vi "Boolean Control - Boolean Button Timed.vi"() -> ()   [LabVIEW 2014]
doc: "Sample numeric display item."
uses:
  <vilib>/NI Veristand/Display Template Support/Display Template Support.llb/cluster_Screen Item Settings.ctl
  <vilib>/NI Veristand/Display Template Support/Display Template Support.llb/cluster_Graph Scale Settings.ctl
  <vilib>/NI Veristand/Display Template Support/Display Template Support.llb/cluster_Graph Plot Settings.ctl
  SubVIs/Boolean Control Timed.ctl
  NationalInstruments.VeriStand.SystemStorage
  <vilib>/NI Veristand/Display Template Support/Display Template Support.llb/enum_Display Template Handler Minimal To Widget Msg.ctl
  <vilib>/NI Veristand/Display Template Support/Display Template Support.llb/enum_Display Template Handler Minimal To Workspace.ctl
  SubVIs/Boolean Control Timed Data.ctl
  <vilib>/NI Veristand/Display Template Support/Display Template Support.llb/sub_Display Template Handler Custom.vi
  <vilib>/NI Veristand/Execution/Workspace/NI VeriStand - Set Single Channel Value.vi
  <vilib>/NI Veristand/Execution/Workspace/NI VeriStand - Get Single Channel Value.vi
  <vilib>/NI Veristand/Execution/Workspace/NI_VS Workspace ExecutionAPI.lvlib
panel:
  in  "NIVS.System Definition Root":refnum<k24>
  in  "NIVS.Gateway IP Address":string
  out "Label":string="Numeric"
  in  "Boolean Timed":T1
  in  "Item.Data":T2
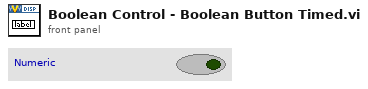
[diagram p1: front panel]
types:
  T1 = typedef "Boolean Control Timed.ctl" = bool
  T2 = typedef "cluster_Screen Item Settings.ctl" = cluster{"Template VI":string, "Position X":i32, "Position Y":i32, "Custom":string, "Show Title Bar":bool, "ID":i32, "Always On Top":bool, "Allow Resize":bool, "Allow Minimize":bool, "Allow Close":bool, "Size to Screen":bool, "Screen.ID":i32, "State":enum16{"Normal", "New"}, "Title":string, "Window Bounds":cluster{"[0]":i16, "[1]":i16, "[2]":i16, "[3]":i16}, "Channel Ref":u64, "Unit":string, "Default Units?":bool, "Flash Limit?":bool, "Color 1":u32, "Color 2":u32, "Color 3":u32, "Color 4":u32, "Bck Color":u32, "Fore Color":u32, "Limit 1":dbl, "Limit 2":dbl, "Limit 3":dbl, "Limit 4":dbl, "Limit Mode 1":i32, "Limit Mode 2":i32, "Limit Mode 3":i32, "Limit Mode 4":i32, "Scale Precision":i32, "Scale Min":dbl, "Scale Max":dbl, "Format":i32, "Precision":i32, "Background Type":i32, "IDs":i32[], "Units":string[], "Labels":string[], "Scale Factor":dbl, "Scale Offset":dbl, "YScale Index":u32[], "XScale":T3, "YScales":T3[], "Plots":T4[], "Update Period":dbl, "History Length":dbl, "My.Ref":refnum<vi>, "Is Control?":bool, "Channel Paths":string[], "Custom Data":variant}
  T3 = typedef "cluster_Graph Scale Settings.ctl" = cluster{"Format":u8, "Precision":u8, "Fit":u8, "Label":string, "Use Default Label":bool, "Label Visible":bool, "Min":dbl, "Max":dbl}
  T4 = typedef "cluster_Graph Plot Settings.ctl" = cluster{"Bar Style":u8, "Fill To":i16, "Fill/PtColor":u32, "Line Style":u8, "Line Width":u8, "Color":u32, "Interp":u8, "Point Style":u8}
  T5 = cluster{"Timer Running?":bool, "Initial Time":u32}
  T6 = typedef "enum_Display Template Handler Minimal To Workspace.ctl" = cluster{"Operation":enum16{"SetCustomData", "DeleteItem"}, "Data":variant}
  T7 = typedef "enum_Display Template Handler Minimal To Widget Msg.ctl" = enum16{"Stop", "LaunchConfigDialog"}
  T8 = typedef "Boolean Control Timed Data.ctl" = cluster{"Node Path":string, "Time (ms)":u32}
  T9 = typedef "NI_VS Workspace ExecutionAPI.lvlib/WorkspaceAPI.ctl" = refnum<k24>
  T10 = typedef "NI_VS Workspace ExecutionAPI.lvlib/SystemState.ctl" = u8
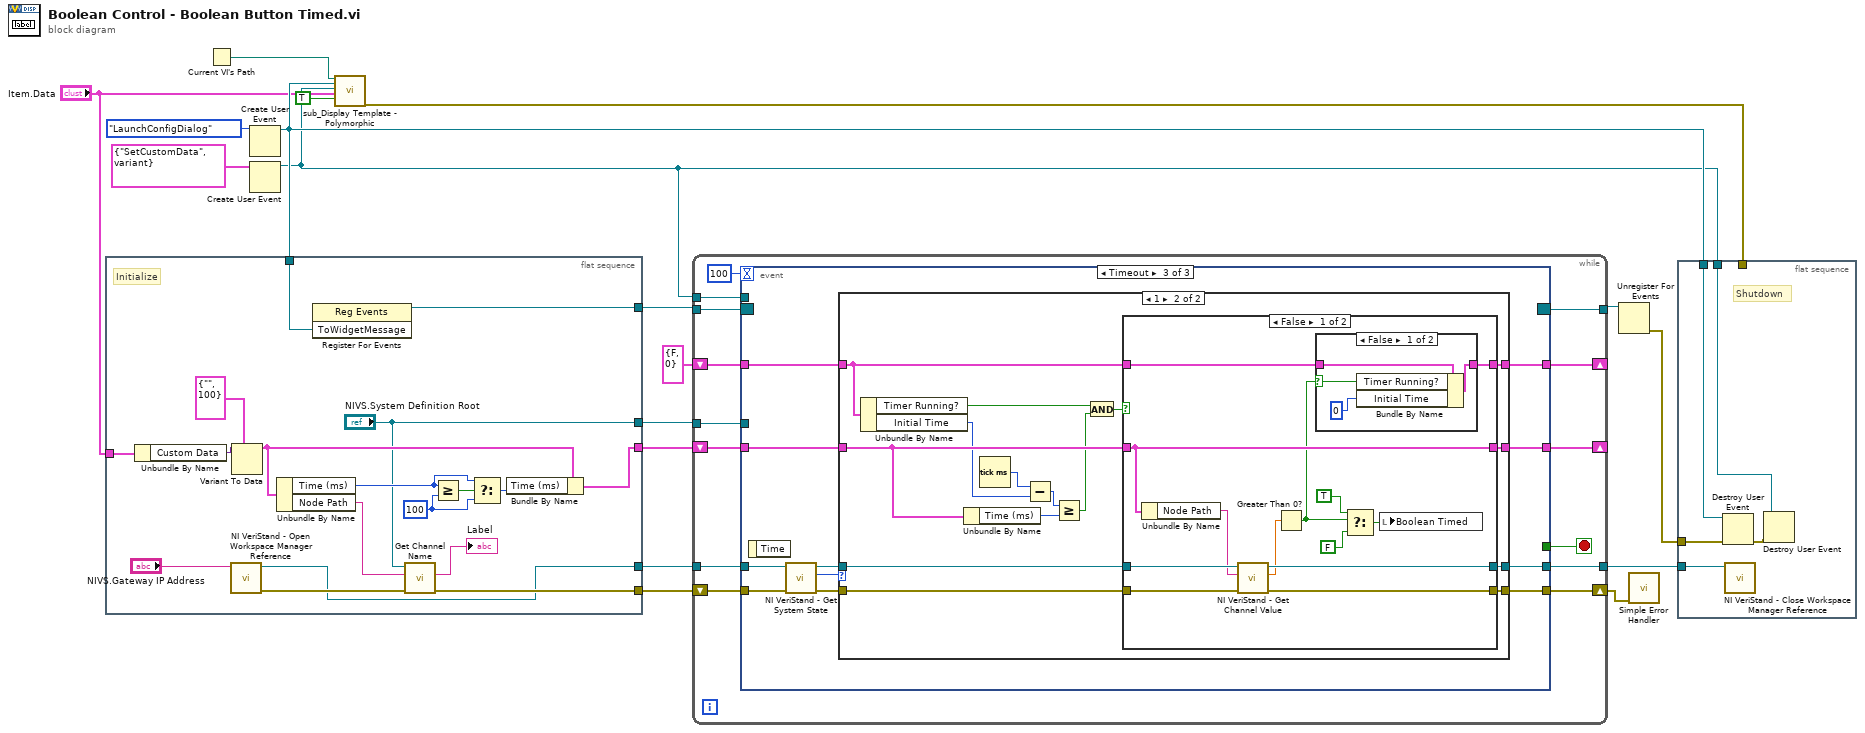
[diagram p0: block diagram]
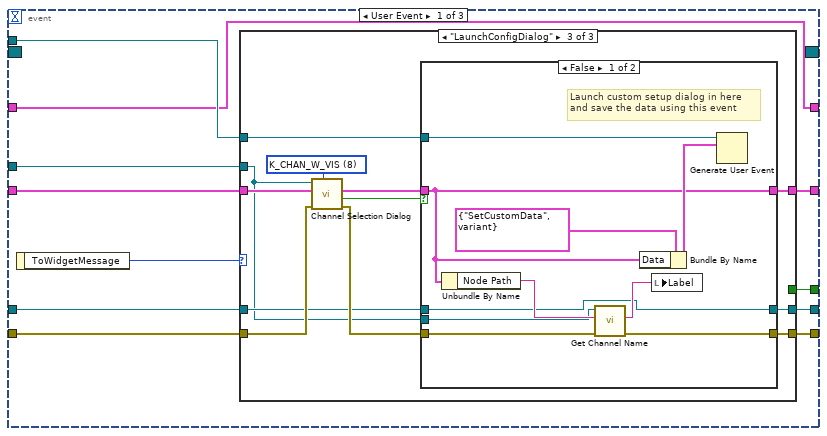
[diagram p2: hidden frame]
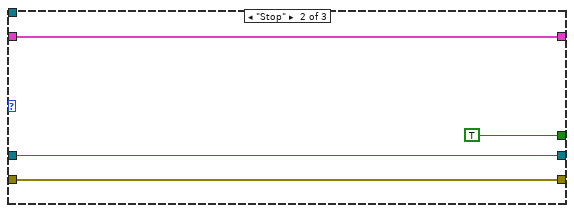
[diagram p4: hidden frame]
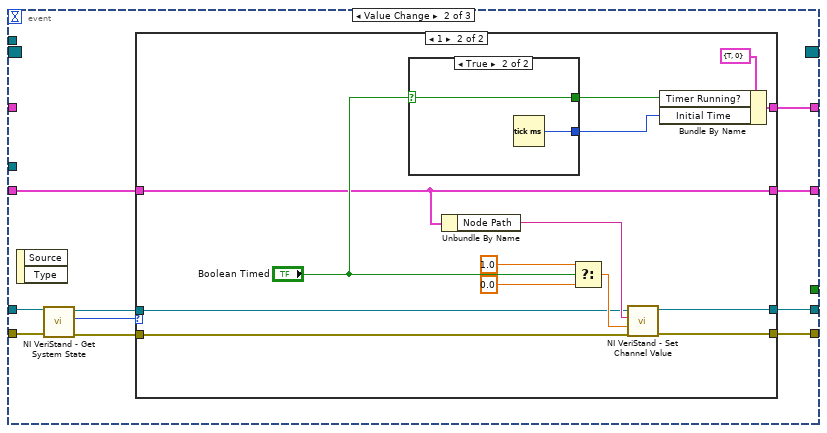
[diagram p6: hidden frame]
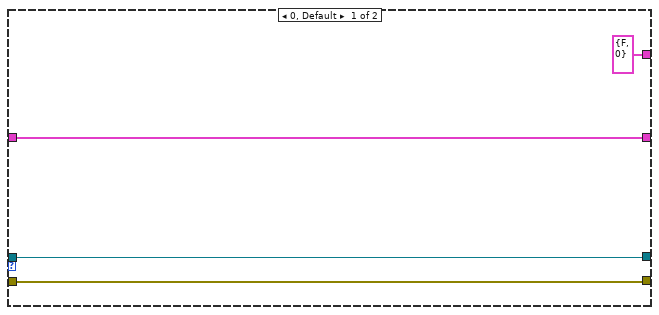
[diagram p7: hidden frame]
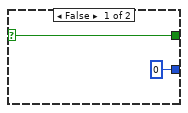
[diagram p8: hidden frame]
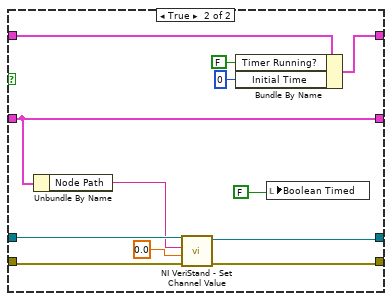
[diagram p11: hidden frame]
diagram:
  n1 = flat-sequence {
    tunnel: [w36] -> w16
    tunnel: w13 -> [w35]
    tunnel: "Item.Data" -> [w34]
    tunnel: [w21] -> w7
    tunnel: [w19] -> w4
    tunnel: [w29] -> w5
    tunnel: ["NIVS.System Definition Root"] -> w6
    frame #0 {
      w23 = u32 100 ("y")
      # "Initialize"
      n2 = Unbundle By Name(w34) -> ("Custom Data"=w33:variant)
      n3 = call <vilib>:"NI VeriStand - Open Workspace Manager Reference.vi"("Gateway IP Address (\"\": localhost)"="NIVS.Gateway IP Address") -> ("error out"=w31:errorcluster, "WorkspaceManager"=w19:T9)  [unwired: 9 in]
      n4 = Variant To Data(type=T8 {"Node Path"="", "Time (ms)"=100}, Variant=w33) -> (data=w26:T8)  [unwired: 1 in, 1 out]
      n5 = Unbundle By Name(w26) -> ("Time (ms)"=w24:u32, "Node Path"=w27:string)
      n6 = register-events(w35) -> (reference out=w36:refnum<event-registration>)  [unwired: 2 in, 1 out]
      n7 = call "Get Channel Name.vi"("error in (no error)"=w31, "Node Path"=w27, "NIVS.System Definition Root in"="NIVS.System Definition Root") -> ("error out"=w29:errorcluster, "Name"=→"Label":string)  [unwired: 6 in, 1 out]
      n8 = Greater Or Equal?(x=w24, y=w23) -> (x >= y?=w25:bool)
      n9 = Select(t=w24, s=w25, f=w23) -> (s? t:f=w22:u32)
      n10 = Bundle By Name(cluster=w26, "Time (ms)"=w22) -> (w21:T8)
    }
  }
  n11 = Current VI's Path() -> (path=w11:path)
  n12 = Create User Event(user event datatype=enum_Display_Template_Handler_Minimal_To_Widget_Msg."LaunchConfigDialog" ("ToWidgetMessage")) -> (user event=w13:refnum<user-event>)  [unwired: 1 in, 1 out]
  n13 = Create User Event(user event datatype=T6 {"Operation"=enum."SetCustomData", "Data"=variant} ("Data")) -> (user event=w9:refnum<user-event>)  [unwired: 1 in, 1 out]
  n14 = call-poly <vilib>:"sub_Display Template - Polymorphic.vi"("Parent.Path"=w11, "ToWidgetEvent"=w13, "ToWorkspace"=w9, "Item.Data"="Item.Data", "Resizable"=TRUE) -> ("error out"=w18:errorcluster)  [unwired: 1 in, 13 out]
  n15 = while {
    tunnel: w16 -> [w50]
    tunnel: [w48] -> w15
    tunnel: w9 -> [w47]
    shift-right: [w40] -> _
    shift-left: w7 -> [w46]
    tunnel: w6 -> [w45]
    shift-right: [w42] -> w1
    shift-left: w5 -> [w44]
    tunnel: w4 -> [w43]
    tunnel: [w41] -> w3
    shift-right: [w38] -> _
    shift-left: T5 {"Timer Running?"=FALSE, "Initial Time"=0} -> [w37]
    stop <- w49 stop-if-true
    n16 = event shown="[2] Timeout" {
      selector: w50 -> [_ _ _]
      dyn-events: [_ _ _] -> w48
      timeout: 100 -> [_ _ _]
      tunnel: [w60 _ _] -> w49
      tunnel: w47 -> [w59 _ _]
      tunnel: w46 -> [w58 w101 w132]
      tunnel: w45 -> [w57 _ _]
      tunnel: w44 -> [w56 w98 w129]
      tunnel: w43 -> [w55 w99 w130]
      tunnel: [w54 w103 w136] -> w42
      tunnel: [w53 w102 w135] -> w41
      tunnel: [w52 w94 w134] -> w40
      tunnel: [w51 w100 w131] -> w38
      tunnel: w37 -> [w51 _ w133]
      event User Event {
        n17 = event-data() -> ("ToWidgetMessage"=w61:T7)  [unwired: 1 out]
        n18 = case shown="\"LaunchConfigDialog\"" w61 {
          tunnel: [_ TRUE _] -> w60
          tunnel: w59 -> [_ _ w80]
          tunnel: w58 -> [w62 w65 w78]
          tunnel: w57 -> [_ _ w69]
          tunnel: w56 -> [w64 w67 w77]
          tunnel: w55 -> [w63 w66 w73]
          tunnel: [w64 w67 w72] -> w54
          tunnel: [w63 w66 w71] -> w53
          tunnel: [w62 w65 w70] -> w52
          frame Default {
          }
          frame "Stop" {
          }
          frame "LaunchConfigDialog" {
            w79 = u8 8 items=["K_CHAN_R", "K_CHAN_W", "K_CHAN_RW", "K_CHAN_VOLT", "K_CHAN_FAULT", "K_ALL", "K_CUSTOM", "K_CHAN_R_VIS", "K_CHAN_W_VIS", "K_CHAN_RW_VIS", "K_CHAN_VOLT_VIS", "K_CHAN_FAULT_VIS"] ("DisplayFilter")
            n19 = call "Channel Selection Dialog.vi"("DisplayFilter"=w79, "error in (no error)"=w77, "Custom Data in"=w78, "NIVS.System Definition Root"=w69) -> ("error out"=w74:errorcluster, "Cancelled"=w76:bool, "Custom Data out"=w75:T8)  [unwired: 5 in]
            n20 = case shown="False" w76 {
              tunnel: w80 -> [w90 _]
              tunnel: w75 -> [w84 w91]
              tunnel: w74 -> [w86 w92]
              tunnel: w73 -> [w82 w93]
              tunnel: [w85 w92] -> w72
              tunnel: [w82 w93] -> w71
              tunnel: [w84 w91] -> w70
              tunnel: w69 -> [w81 _]
              frame False {
                # "Launch custom setup dialog in here\nand save the data using this event"
                n21 = Unbundle By Name(w84) -> ("Node Path"=w83:string)
                n22 = call "Get Channel Name.vi"("error in (no error)"=w86, "Node Path"=w83, "NIVS.System Definition Root in"=w81) -> ("error out"=w85:errorcluster, "Name"=w87:string)  [unwired: 6 in, 1 out]
                n23 = Bundle By Name(cluster=T6 {"Operation"=enum."SetCustomData", "Data"=variant} ("event data"), "Data"=w84) -> (w88:T6)
                n24 = local write "Label"(w87) -> ()
                n25 = Generate User Event(user event=w90, event data cluster=w88) -> ()  [unwired: 2 in, 2 out]
              }
              frame True {
              }
            }
          }
        }
      }
      event Value Change {
        n26 = event-data() -> ()  [unwired: 3 out]
        n27 = call <vilib>:"NI VeriStand - Get System State.vi"("error in (no error)"=w98, "WorkspaceManager in"=w99) -> ("error out"=w97:errorcluster, "System State"=w95:T10, "WorkspaceManager  out"=w96:T9)  [unwired: 5 in, 2 out]
        n28 = case shown="1" w95 {
          tunnel: [w107 w121] -> w103
          tunnel: [w106 w120] -> w102
          tunnel: w101 -> [w105 w108]
          tunnel: [T5 {"Timer Running?"=FALSE, "Initial Time"=0} w111] -> w100
          tunnel: w97 -> [w107 w110]
          tunnel: w96 -> [w106 w109]
          tunnel: [w105 w108] -> w94
          frame 0, Default {
          }
          frame 1 {
            n29 = case shown="True" "Boolean Timed" {
              selector: "Boolean Timed" -> [w123 w125]
              tunnel: [w123 w125] -> w113
              tunnel: [u32 0 ("millisecond timer value") w124] -> w112
              frame False {
              }
              frame True {
                n30 = Tick Count (ms)() -> (millisecond timer value=w124:u32)
              }
            }
            n31 = Unbundle By Name(w108) -> ("Node Path"=w116:string)
            n32 = Select(t=1.0, s="Boolean Timed", f=0.0) -> (s? t:f=w117:dbl)
            n33 = call-poly <vilib>:"NI VeriStand - Set Channel Value.vi"("error in (no error)"=w110, "Value"=w117, "Channel"=w116, "WorkspaceManager in"=w109) -> ("error out"=w121:errorcluster, "WorkspaceManager out"=w120:T9)  [unwired: 6 in]
            n34 = Bundle By Name(cluster=T5 {"Timer Running?"=TRUE, "Initial Time"=0}, "Timer Running?"=w113, "Initial Time"=w112) -> (w111:T5)
          }
        }
      }
      event Timeout {
        n35 = event-data() -> ()  [unwired: 2 out]
        n36 = call <vilib>:"NI VeriStand - Get System State.vi"("error in (no error)"=w129, "WorkspaceManager in"=w130) -> ("error out"=w128:errorcluster, "System State"=w126:T10, "WorkspaceManager  out"=w127:T9)  [unwired: 5 in, 2 out]
        n37 = case shown="1" w126 {
          tunnel: [w137 w155] -> w136
          tunnel: [w138 w154] -> w135
          tunnel: [w139 w153] -> w134
          tunnel: w133 -> [w140 w152]
          tunnel: w132 -> [w139 w148]
          tunnel: [w140 w143] -> w131
          tunnel: w128 -> [w137 w142]
          tunnel: w127 -> [w138 w141]
          frame 0, Default {
          }
          frame 1 {
            n38 = Unbundle By Name(w152) -> ("Timer Running?"=w145:bool, "Initial Time"=w147:u32)
            n39 = Unbundle By Name(w148) -> ("Time (ms)"=w150:u32)
            n40 = Tick Count (ms)() -> (millisecond timer value=w151:u32)
            n41 = Subtract(x=w151, y=w147) -> (x-y=w149:u32)
            n42 = Greater Or Equal?(x=w149, y=w150) -> (x >= y?=w146:bool)
            n43 = And(x=w145, y=w146) -> (x .and. y?=w144:bool)
            n44 = case shown="False" w144 {
              tunnel: w142 -> [w168 w184]
              tunnel: w141 -> [w167 w185]
              tunnel: [w166 w182] -> w155
              tunnel: [w165 w183] -> w154
              tunnel: w148 -> [w159 w179]
              tunnel: [w159 w179] -> w153
              tunnel: w152 -> [w157 w178]
              tunnel: [w156 w175] -> w143
              frame False {
                n45 = Unbundle By Name(w159) -> ("Node Path"=w160:string)
                n46 = call-poly <vilib>:"NI VeriStand - Get Channel Value.vi"("error in (no error)"=w168, "Channel"=w160, "WorkspaceManager in"=w167) -> ("error out"=w166:errorcluster, "Value"=w164:dbl, "WorkspaceManager out"=w165:T9)  [unwired: 6 in]
                n47 = Greater Than 0?(x=w164) -> (x > 0?=w158:bool)
                n48 = case shown="False" w158 {
                  selector: w158 -> [w171 _]
                  tunnel: w157 -> [w172 w173]
                  tunnel: [w169 w173] -> w156
                  frame False {
                    n49 = Bundle By Name(cluster=w172, "Timer Running?"=w171, "Initial Time"=u32 0) -> (w169:T5)
                  }
                  frame True {
                  }
                }
                n50 = Select(t=TRUE, s=w158, f=FALSE) -> (s? t:f=w161:bool)
                n51 = local write "Boolean Timed"(w161) -> ()
              }
              frame True {
                n52 = Unbundle By Name(w179) -> ("Node Path"=w181:string)
                n53 = call-poly <vilib>:"NI VeriStand - Set Channel Value.vi"("error in (no error)"=w184, "Value"=0.0, "Channel"=w181, "WorkspaceManager in"=w185) -> ("error out"=w182:errorcluster, "WorkspaceManager out"=w183:T9)  [unwired: 6 in]
                n54 = Bundle By Name(cluster=w178, "Timer Running?"=FALSE, "Initial Time"=u32 0) -> (w175:T5)
                n55 = local write "Boolean Timed"(FALSE) -> ()
              }
            }
          }
        }
      }
    }
  }
  n56 = Unregister For Events(event registration refnum=w15) -> (error out=w14:errorcluster)  [unwired: 1 in]
  n57 = call <vilib>:"Simple Error Handler.vi"("error in (no error)"=w1) -> ()  [unwired: 4 in, 5 out]
  n58 = flat-sequence {
    tunnel: w18 -> [_]
    tunnel: w14 -> [w189]
    tunnel: w13 -> [w190]
    tunnel: w9 -> [w187]
    tunnel: w3 -> [w186]
    frame #0 {
      # "Shutdown"
      n59 = Destroy User Event(user event=w190, error in=w189) -> (error out=w188:errorcluster)
      n60 = call <vilib>:"NI VeriStand - Close Workspace Manager Reference.vi"("WorkspaceManager"=w186) -> ()  [unwired: 10 in, 1 out]
      n61 = Destroy User Event(user event=w187, error in=w188) -> ()  [unwired: 1 out]
    }
  }
